vi "IMU_Initialize_Data.vi"(8 "error in (no error)":errorcluster caption="Fehler (Eingang, kein Fehler)", 11 "MultiWii Data Cluster":refnum<vi>) -> (0 "error out":errorcluster caption="Fehler (Ausgang)")   [LabVIEW 2017]
uses:
  IMU_Data_Cluster.ctl
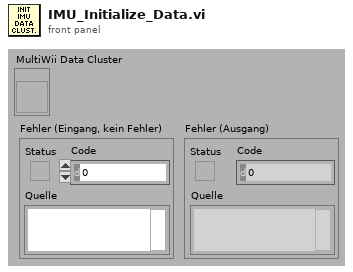
[diagram p1: front panel]
types:
  T1 = typedef "IMU_Data_Cluster.ctl" = cluster{"Firmware Revision":string, "Multitype Name":string, "Cycle Time":u16, "I²C Error Count":u16, "ACC present":bool, "Baro present":bool, "Mag Present":bool, "GPS present":bool, "Sonar present":bool, "Acc X axis (Roll)":dbl, "Acc Y axis (Pitch)":dbl, "Acc Z axis (Yaw)":dbl, "Gyro X axis (Roll)":dbl, "Gyro Y axis (Pitch)":dbl, "Gyro Z axis (Yaw)":dbl, "Mag X axis (Roll)":dbl, "Mag Y axis (Pitch)":dbl, "Mag Z axis (Yaw)":dbl, "X angle (Roll)":dbl, "Y angle (Pitch)":dbl, "Heading [°]":dbl, "Altitude [m]":dbl, "Vario":dbl, "GPS_Fix":u8, "GPS_NumSat":u8, "GPS_coord[LAT]":dbl, "GPS_coord[LON]":dbl, "GPS_Altitude":dbl, "GPS_Speed over Ground":dbl, "GPS_Ground Course":dbl, "Baro P [mbara]":dbl, "Baro T [°C]":dbl, "Altitude abs [m]":dbl}
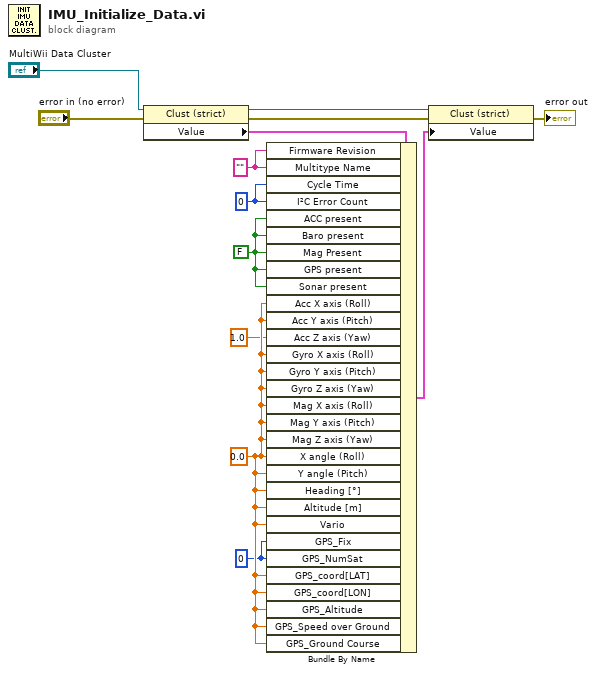
[diagram p0: block diagram]
diagram:
  w9 = u8 0 ("Cycle Time")
  w10 = 0.0 ("Acc X axis (Roll)")
  w11 = FALSE ("ACC present")
  w12 = u16 0 ("Cycle Time")
  w13 = "" ("Firmware Revision")
  n1 = property class="Clust (strict)"(reference="MultiWii Data Cluster", error in="error in (no error)") -> (reference out=w4:refnum<vi>, error out=w1:errorcluster, "Value"=w6:T1)
  n2 = Bundle By Name(cluster=w6, "Firmware Revision"=w13, "Multitype Name"=w13, "Cycle Time"=w12, "I²C Error Count"=w12, "ACC present"=w11, "Baro present"=w11, "Mag Present"=w11, "GPS present"=w11, "Sonar present"=w11, "Acc X axis (Roll)"=w10, "Acc Y axis (Pitch)"=w10, "Acc Z axis (Yaw)"=1.0, "Gyro X axis (Roll)"=w10, "Gyro Y axis (Pitch)"=w10, "Gyro Z axis (Yaw)"=w10, "Mag X axis (Roll)"=w10, "Mag Y axis (Pitch)"=w10, "Mag Z axis (Yaw)"=w10, "X angle (Roll)"=w10, "Y angle (Pitch)"=w10, "Heading [°]"=w10, "Altitude [m]"=w10, "Vario"=w10, "GPS_Fix"=w9, "GPS_NumSat"=w9, "GPS_coord[LAT]"=w10, "GPS_coord[LON]"=w10, "GPS_Altitude"=w10, "GPS_Speed over Ground"=w10, "GPS_Ground Course"=w10) -> (w7:T1)
  n3 = property class="Clust (strict)"(reference=w4, error in=w1, "Value"=w7) -> (error out=→"error out":errorcluster)  [unwired: 1 out]
